vi "Psense.vi"() -> ()   [LabVIEW 2015]
uses:
  <vilib>/myRIO/Instrument Drivers/Onboard IO/I2C/typedefs/I2C User Configuration.ctl
  <vilib>/myRIO/Instrument Drivers/Onboard IO/I2C/typedefs/I2C Transfer Rate.ctl
  <vilib>/Platform/TimedLoop/XDataNode/timing_clust.ctl
  <vilib>/Platform/TimedLoop/XDataNode/nitl_modes.ctl
  <vilib>/Platform/TimedLoop/XDataNode/wakeup.ctl
  <vilib>/myRIO/Common/Instrument Driver Framework/myRIO v1.0/UART/vis/myRIO v1.0 Close UART.vi
  <vilib>/Utility/error.llb/Error Cluster From Error Code.vi
  <vilib>/myRIO/Common/Instrument Driver Framework/myRIO v1.0/I2C/vis/myRIO v1.0 Configure I2C.vi
  <vilib>/myRIO/Common/Instrument Driver Framework/myRIO v1.0/I2C/vis/myRIO v1.0 Write I2C.vi
  <vilib>/myRIO/Common/Instrument Driver Framework/myRIO v1.0/I2C/vis/myRIO v1.0 Read I2C.vi
  <vilib>/myRIO/Common/Instrument Driver Framework/Utilities/vis/FPGA Ref Manager.vi
  <vilib>/myRIO/Common/Instrument Driver Framework/myRIO v1.0/myRIO v1.0 Reset FPGA.vi
  <vilib>/myRIO/Common/Instrument Driver Framework/myRIO v1.0/IRQ/vis/myRIO v1.0 IRQ Info FGV.vi
  <vilib>/myRIO/Common/Instrument Driver Framework/myRIO v1.0/IRQ/vis/myRIO v1.0 Timer IRQ Info FGV.vi
  <vilib>/myRIO/Common/Instrument Driver Framework/myRIO v1.0/IRQ/vis/myRIO v1.0 ISR Agent.vi
  <vilib>/platform/TimedLoop/XDataNode/XDataNode.xnode
  <vilib>/myRIO/Instrument Drivers/Onboard IO/I2C/I2C.lvlib
  <vilib>/Platform/TimedLoop/XDataNode/XDNodeRunTimeDep.lvlib
  <vilib>/myRIO/Instrument Drivers/Utilities/Utilities.lvlib
panel:
  out "P":i32
  out "Pressure":i32(slide) scale=0.0..10.0
  out "T":dbl(knob) scale=20.0..30.0
  out "T":u32
  out "Pressure":u32
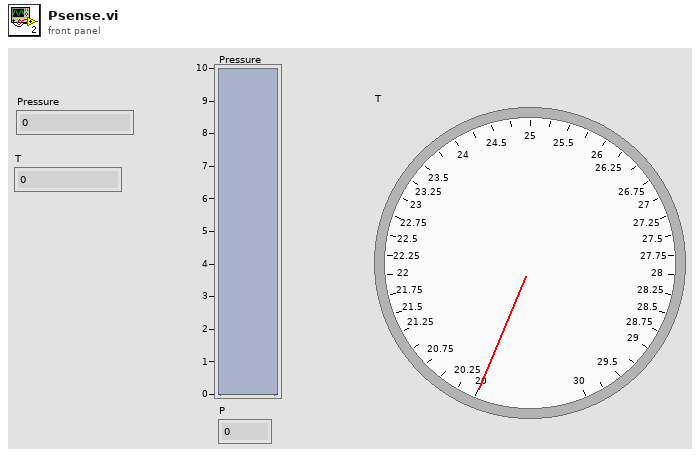
[diagram p1: front panel]
types:
  T1 = typedef "I2C.lvlib/I2C User Configuration.ctl" = cluster{"I2C Transfer Rate":T2}
  T2 = typedef "I2C.lvlib/I2C Transfer Rate.ctl" = enum16{"Standard mode (100 kbps)", "Fast mode (400 kbps)"}
  T3 = typedef "I2C.lvlib/I2C Reference.ctl" = cluster{"myRIO Reference":T4, "I2C Channels Enum":T8, "I2C Configuration":T9}
  T4 = typedef "myRIO Generic Hardware Reference.ctl" = cluster{"myRIO Model":T5, "myRIO Hardware Reference":T6}
  T5 = typedef "Hardware Version Enum.ctl" = enum16{"Unknown", "myRIO-1900", "myRIO-1950", "roboRIO"}
  T6 = typedef "myRIO v1.0 Reference.ctl" = cluster{"Generic FPGA Reference":T7, "Allow multiple opens":bool}
  T7 = typedef "Generic FPGA Reference.ctl" = refnum<k20>
  T8 = typedef "I2C Channels Enum.ctl" = enum16{"Not Connected", "A/I2C", "B/I2C", "I2C/I2C"}
  T9 = typedef "I2C.lvlib/I2C Configuration.ctl" = cluster{"I2C Transfer Rate":T2}
  T10 = typedef "XDNodeRunTimeDep.lvlib/timing_clust.ctl" = cluster{"Expected End [f-1]":u64, "Actual End [f-1]":u64, "Finished Late? [f-1]":bool, "Expected End [i-1]":u64, "Actual End [i-1]":u64, "Finished Late? [i-1]":bool, "Expected Start [i]":u64, "Actual Start [i]":u64, "Expected Start [f]":u64, "Actual Start [f]":u64, "Source Name":string, "Structure Name":string, "Period":i64, "Deadline":i64, "Offset":i64, "Start":i64, "Priority":i32, "Timeout":i32, "Mode":T11, "Wakeup Reason":T12, "Error":errorcluster, "Source Type":string, "Secondary Source Type":string, "Global End Time":u64, "Global Start Time":u64, "Frame Duration":u64, "Iteration Duration":u64, "Assigned CPU":i32, "I/O Scan Engine Mode":u32}
  T11 = typedef "XDNodeRunTimeDep.lvlib/nitl_modes.ctl" = enum32{"No Change", "Process missed periods, maintain original phase", "Discard missed periods, maintain original phase", "Process missed periods, ignore original phase", "Discard missed periods, ignore original phase"}
  T12 = typedef "XDNodeRunTimeDep.lvlib/wakeup.ctl" = enum32{"Normal", "Aborted", "Asynchronous wakeup", "Timing source error", "Timed loop error", "Timeout"}
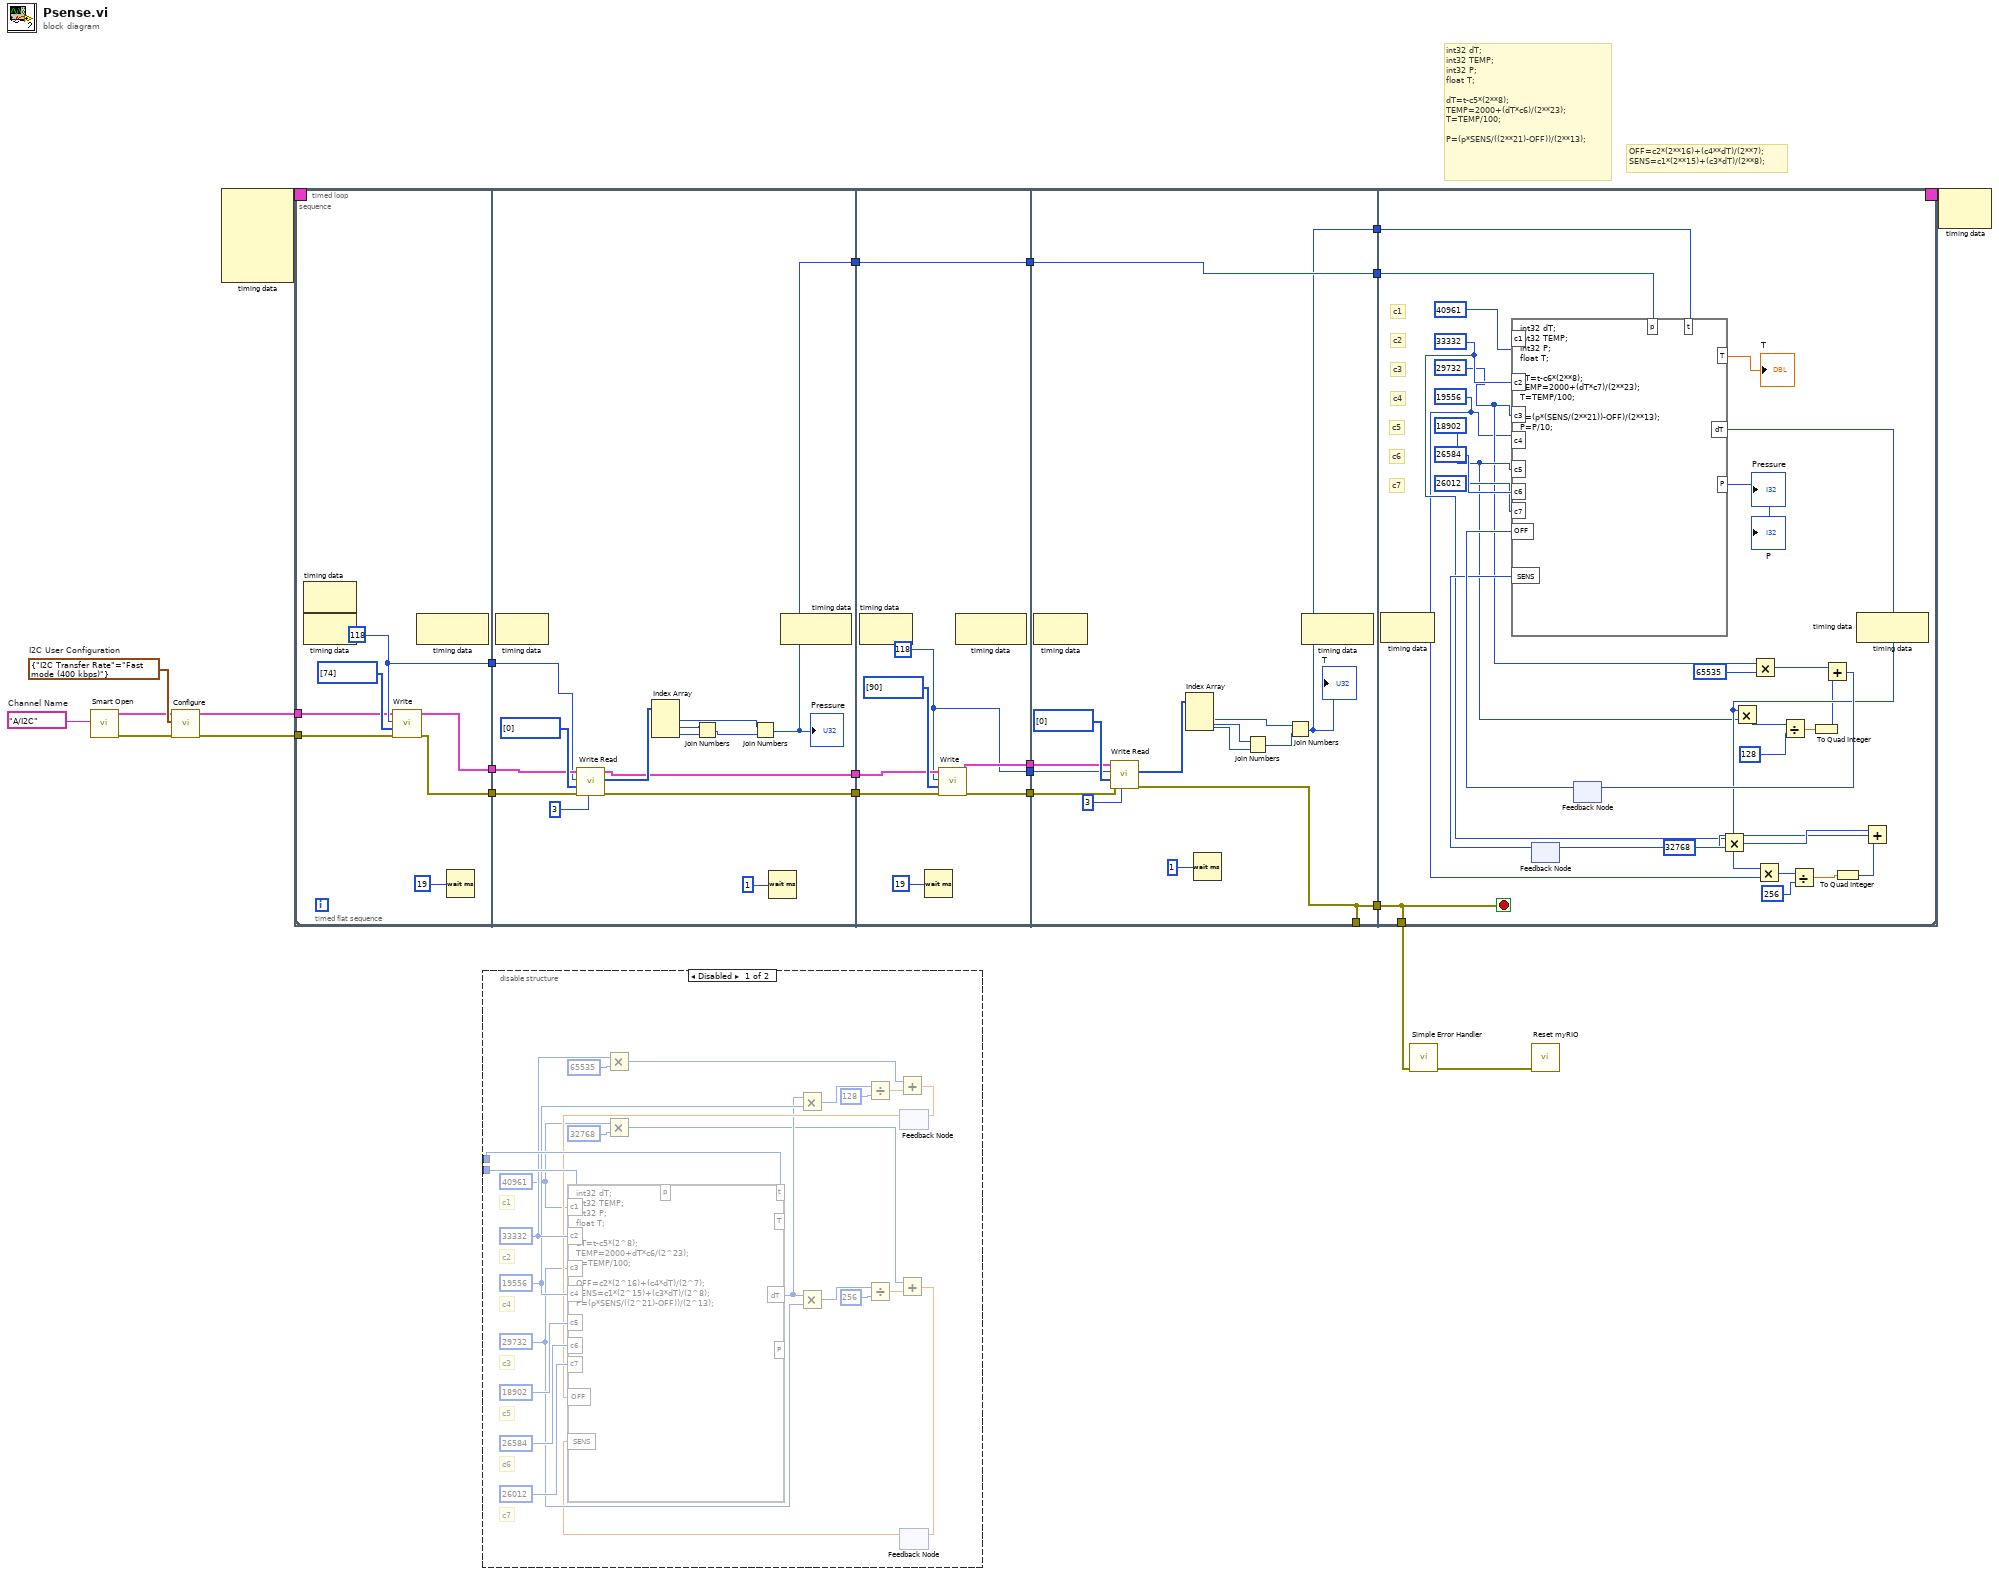
[diagram p0: block diagram]
diagram:
  w9 = T1 {"I2C Transfer Rate"=enum."Fast mode (400 kbps)"}  # I2C User Configuration
  w10 = tag "A/I2C"  # Channel Name
  # "OFF=c2*(2**16)+(c4**dT)/(2**7);\nSENS=c1*(2**15)+(c3*dT)/(2**8);"
  # "int32 dT;\nint32 TEMP;\nint32 P;\nfloat T;\n\ndT=t-c5*(2**8);\nTEMP=2000+(dT*c6)/(2**23);\nT=TEMP/100;\n\nP=(p*SENS/((2**21)-OFF))/(2**13);"
  n1 = call <vilib>:"Smart Open.vi"("Channel Name"=w10) -> ("error out"=w7:errorcluster, "I2C Ref Out"=w8:T3)  [unwired: 9 in]
  n2 = call <vilib>:"Configure.vi"("error in (no error)"=w7, "I2C User Configuration"=w9, "I2C Ref In"=w8) -> ("error out"=w3:errorcluster, "I2C Ref Out"=w4:T3)  [unwired: 7 in]
  n3 = node-c288() -> (w6:T10)  [unwired: 5 in]
  n4 = timed-loop {
    timing: w6 -> [_]
    timing-out: [_] -> w5
    tunnel: [w14] -> _
    tunnel: w4 -> [w13]
    tunnel: w3 -> [w12]
    tunnel: [w11] -> w1
    stop <- w89 stop-if-true
    n5 = timed-sequence {
      timing: _ -> [_]
      timing-out: _ -> [_]
      tunnel: [w23] -> w14
      tunnel: w13 -> [w22]
      tunnel: w12 -> [w21]
      tunnel: [w16] -> w11
      n6 = timed-flat-sequence {
        tunnel: [w37] -> w31
        tunnel: [w36] -> w30
        tunnel: [w35] -> w29
        tunnel: w22 -> [w33]
        tunnel: w21 -> [w32]
        tunnel: w31 -> [w51]
        tunnel: w30 -> [w50]
        tunnel: w29 -> [w49]
        tunnel: [w48] -> w28
        tunnel: [w47] -> w27
        tunnel: [w45] -> w17
        tunnel: w28 -> [w63]
        tunnel: w27 -> [w62]
        tunnel: [w60] -> w26
        tunnel: [w59] -> w25
        tunnel: [w58] -> w24
        tunnel: [w57] -> w18
        tunnel: w17 -> [w57]
        tunnel: w26 -> [w76]
        tunnel: w25 -> [w75]
        tunnel: w24 -> [w74]
        tunnel: [w72] -> w23
        tunnel: [w72] -> w20
        tunnel: [w71] -> w19
        tunnel: w18 -> [w71]
        tunnel: [w67] -> w15
        tunnel: w20 -> [w89]
        tunnel: w19 -> [w94]
        tunnel: [w89] -> w16
        tunnel: w15 -> [w88]
        frame #0 {
          w35 = u8 118 ("Slave Address (7-bit)")
          n7 = node-c288() -> ()  [unwired: 1 in, 1 out]
          n8 = call <vilib>:"Write.vi"("error in (no error)"=w32, "Bytes to Write"=u8[] [74], "Slave Address (7-bit)"=w35, "I2C Ref In"=w33) -> ("error out"=w36:errorcluster, "I2C Ref Out"=w37:T3)  [unwired: 6 in]
          n9 = node-c288() -> ()  [unwired: 1 in, 1 out]
          n10 = Wait (ms)(milliseconds to wait=u32 19) -> ()  [unwired: 1 out]
        }
        frame #1 {
          n11 = node-c288() -> ()  [unwired: 1 in, 1 out]
          n12 = call <vilib>:"Write Read.vi"("Byte Count"=u32 3, "error in (no error)"=w50, "Bytes to Write"=u8[] [0], "Slave Address (7-bit)"=w49, "I2C Ref In"=w51) -> ("error out"=w48:errorcluster, "Bytes Read"=w52:u8[], "I2C Ref Out"=w47:T3)  [unwired: 3 in]
          n13 = Index Array "Index Array"(array=w52) -> (element #1=w41:u8, element #2=w43:u8, element #3=w44:u8)  [unwired: 3 in]
          n14 = Join Numbers(hi=w43, lo=w44) -> ((hi.lo)=w42:u16)
          n15 = Join Numbers(hi=w41, lo=w42) -> ((hi.lo)=w45:u32)
          "Pressure" <- w45
          n16 = Wait (ms)(milliseconds to wait=u32 1) -> ()  [unwired: 1 out]
          n17 = node-c288() -> ()  [unwired: 1 in, 1 out]
        }
        frame #2 {
          w58 = u8 118 ("Slave Address (7-bit)")
          n18 = node-c288() -> ()  [unwired: 1 in, 1 out]
          n19 = Wait (ms)(milliseconds to wait=u32 19) -> ()  [unwired: 1 out]
          n20 = call <vilib>:"Write.vi"("error in (no error)"=w63, "Bytes to Write"=u8[] [90], "Slave Address (7-bit)"=w58, "I2C Ref In"=w62) -> ("error out"=w59:errorcluster, "I2C Ref Out"=w60:T3)  [unwired: 6 in]
          n21 = node-c288() -> ()  [unwired: 1 in, 1 out]
        }
        frame #3 {
          n22 = node-c288() -> ()  [unwired: 1 in, 1 out]
          n23 = call <vilib>:"Write Read.vi"("Byte Count"=u32 3, "error in (no error)"=w75, "Bytes to Write"=u8[] [0], "Slave Address (7-bit)"=w74, "I2C Ref In"=w76) -> ("error out"=w72:errorcluster, "Bytes Read"=w78:u8[])  [unwired: 3 in, 1 out]
          n24 = Index Array "Index Array"(array=w78) -> (element #1=w68:u8, element #2=w69:u8, element #3=w70:u8)  [unwired: 3 in]
          n25 = Wait (ms)(milliseconds to wait=u32 1) -> ()  [unwired: 1 out]
          n26 = Join Numbers(hi=w69, lo=w70) -> ((hi.lo)=w77:u16)
          n27 = Join Numbers(hi=w68, lo=w77) -> ((hi.lo)=w67:u32)
          "T" <- w67
          n28 = node-c288() -> ()  [unwired: 1 in, 1 out]
        }
        frame #4 {
          w85 = u16 33332 ("Slave Address (7-bit)")
          w87 = i16 18902 ("Byte Count")
          w83 = i16 19556 ("Byte Count")
          w84 = i16 29732 ("Byte Count")
          # "c7"
          # "c6"
          # "c5"
          # "c4"
          # "c3"
          # "c2"
          # "c1"
          n29 = node-c288() -> ()  [unwired: 1 in, 1 out]
          n30 = feedback #1() -> (w96:i64)  [unwired: 1 in]
          n31 = feedback #2() -> (w103:i64)  [unwired: 1 in]
          n32 = formula code="int32 dT;\nint32 TEMP;\nint32 P;\nfloat T;\n\ndT=t-c6*(2**8);\nTEMP=2000+(dT*c7)/(2**23);\nT=TEMP/100;\n\nP=(p*(SENS/(2**21))-OFF)/(2**13);\nP=P/10;"("c1"=u16 40961 ("Byte Count"), "c2"=w85, "c3"=w84, "c4"=w83, "c5"=w87, "c6"=i16 26584 ("Byte Count"), "c7"=i16 26012 ("Byte Count"), "p"=w94, "t"=w88, "OFF"=w103, "SENS"=w96) -> ("T"=→"T":dbl, "dT"=w101:i32, "P"=→"Pressure" →"P":i32)
          n33 = Multiply(x=w85, y=u16 32768) -> (x*y=w98:u16)
          n34 = Multiply(x=w101, y=w87) -> (x*y=w106:i32)
          n35 = Multiply(x=w84, y=u16 65535) -> (x*y=w107:u16)
          n36 = Multiply(x=w101, y=w83) -> (x*y=w100:i32)
          n37 = Divide(x=w106, y=u16 128) -> (x/y=w93:dbl)
          n38 = Divide(x=w100, y=u16 256) -> (x/y=w91:dbl)
          n39 = To Quad Integer(1:w93) -> (0:w92:i64)
          n40 = Add(x=w107, y=w92) -> (x+y=w104:i64)
          n41 = feedback-in #2(w104) -> ()
          n42 = To Quad Integer(1:w91) -> (0:w90:i64)
          n43 = node-c288() -> ()  [unwired: 1 in, 1 out]
          n44 = Add(x=w98, y=w90) -> (x+y=w97:i64)
          n45 = feedback-in #1(w97) -> ()
        }
      }
    }
    n46 = node-c288() -> ()  [unwired: 1 in, 1 out]
    n47 = node-c288() -> ()  [unwired: 1 in, 1 out]
  }
  n48 = disable-structure shown="Disabled" {
    disable-tunnel: _ -> [w138 _]
    disable-tunnel: _ -> [w137 _]
    frame Disabled {
      w135 = u16 33332 ("Slave Address (7-bit)")
      w132 = i16 19556 ("Byte Count")
      w123 = i16 29732 ("Byte Count")
      w125 = u16 40961 ("Byte Count")
      # "c7"
      # "c6"
      # "c5"
      # "c4"
      # "c3"
      # "c2"
      # "c1"
      n49 = Multiply(x=w135, y=u16 65535) -> (x*y=w133:u16)
      n50 = Multiply(x=w125, y=u16 32768) -> (x*y=w120:u16)
      n51 = feedback #3() -> (w127:dbl)  [unwired: 1 in]
      n52 = feedback #4() -> (w117:dbl)  [unwired: 1 in]
      n53 = formula code="int32 dT;\nint32 TEMP;\nint32 P;\nfloat T;\n\ndT=t-c5*(2^8);\nTEMP=2000+dT*c6/(2^23);\nT=TEMP/100;\n\nOFF=c2*(2^16)+(c4*dT)/(2^7);\nSENS=c1*(2^15)+(c3*dT)/(2^8);\nP=(p*SENS/((2^21)-OFF))/(2^13);"("c1"=w125, "c2"=w135, "c3"=w123, "c4"=w132, "c5"=i16 18902 ("Byte Count"), "c6"=i16 26584 ("Byte Count"), "c7"=i16 26012 ("Byte Count"), "p"=w138, "t"=w137, "OFF"=w127, "SENS"=w117) -> ("T"=w136:dbl, "dT"=w124:i32, "P"=w116:i32)
      n54 = Multiply(x=w124, y=w132) -> (x*y=w131:i32)
      n55 = Multiply(x=w124, y=w123) -> (x*y=w122:i32)
      n56 = Divide(x=w131, y=u16 128) -> (x/y=w129:dbl)
      n57 = Divide(x=w122, y=u16 256) -> (x/y=w119:dbl)
      n58 = Add(x=w133, y=w129) -> (x+y=w128:dbl)
      n59 = Add(x=w120, y=w119) -> (x+y=w118:dbl)
      n60 = feedback-in #3(w128) -> ()
      n61 = feedback-in #4(w118) -> ()
    }
    frame Enabled {
    }
  }
  n62 = call <vilib>:"Simple Error Handler.vi"("error in (no error)"=w1) -> ("error out"=w2:errorcluster)  [unwired: 4 in, 4 out]
  n63 = call <vilib>:"Reset myRIO.vi"("error in (no error)"=w2) -> ()  [unwired: 10 in, 1 out]
  n64 = node-c288(w5) -> ()  [unwired: 1 out]
